vi "nanocal -- nuclear schottky goodness V2.vi"(0 "ζ":dbl(slide)=0.23496699999999998 min=0.0 max=0.3 step=1e-06 scale=0.01..10.0 scale format="%#_3p", 1 "T1":dbl(slide)=0.26762 min=0.0 max=0.3 step=1e-06 scale=0.001..10.0 scale format="%#_3p", 2 "τS":dbl(slide)=0.24445899999999998 min=0.0 max=0.3 step=1e-06 scale=0.001..10.0 scale format="%#_3p", 3 "τN":dbl(slide)=2.349673 min=0.0 max=0.3 step=1e-06 scale=0.001..10.0 scale format="%#_3p", 4 "τC":dbl(slide)=0.0059759999999999995 min=0.0 max=0.3 step=1e-06 scale=0.001..10.0 scale format="%#_3p", 5 "κ0":dbl(slide)=5.58e-10 min=0.0 max=0.3 step=1e-12 scale=1e-10..1e-06 scale format="%#_3p", 7 "ω (rad/sec)":dbl[](array[numeric])=[32012.991918577427, 32390.261658505893, 32466.39798177853, 32499.14340521798, 32517.39286113775, 32529.046092051318, 32537.14525712326, 32543.111142615544, 32547.696343954158, 32551.33675949651, 32554.302325209504, 32556.769142360055, 32558.856995237307, 32560.650202739795, 32562.209843476354, 32563.58125099723, 32564.7987833122, 32565.88895894197, 32566.872575330308, 32567.766175404246, 32568.583086316496, 32569.334166794306, 32570.02835688638, 32570.673085530187, 32571.274580490695, 32571.838104118455, 32572.36813539066, 32572.868514009202, 32573.342552524307, 32573.793126289274, 32574.222746575288, 32574.633618125405, 32575.027687968828, 32575.40668442971, 32575.772149741057, 32576.12546690325, 32576.467883345118, 32576.800529469096, 32577.124435064776, 32577.440543590797, 32577.749724325146, 32578.052781957467, 32578.35046682089, 32578.643482565894, 32578.932492128843, 32579.218126471686, 32579.500987779396, 32579.781656707495, 32580.06069600583, 32580.338656060805, 32580.616078519142, 32580.89350097748, 32581.171461032456, 32581.45050033079, 32581.73116925889, 32582.0140305666, 32582.29966469628, 32582.58867447239, 32582.88169000423, 32583.179375080817, 32583.48243271314, 32583.791613234323, 32584.10772197351, 32584.43162756919, 32584.764273480003, 32585.106690135035, 32585.460007297228, 32585.825472395412, 32586.204468856296, 32586.59853891288, 32587.009410462997, 32587.439030535847, 32587.889604513977, 32588.363642815923, 32588.86402143446, 32589.39405291983, 32589.957576334426, 32590.559071508098, 32591.203800151903, 32591.897990030815, 32592.64907072179, 32593.46598163404, 32594.359581707977, 32595.343197883154, 32596.433373726086, 32597.650906041054, 32599.022313348767, 32600.58195429849, 32602.375161800977, 32604.46301467823, 32606.929831615616, 32609.895397541775, 32613.535812870963, 32618.12101442274, 32624.086899701866, 32632.186064986967, 32643.839295900536, 32662.088751820305, 32694.834175046595, 32770.97049853239], 8 "weighting strategy":T1, 9 "Voltage IN (V)":cdb[](array[numeric])=[1.7183506006211996e-05+0.0i, 1.7124360968751133e-05+0.0i, 1.7049104347380084e-05+0.0i, 1.700437896335042e-05+0.0i, 1.6984579723285106e-05+0.0i, 1.702277369054923e-05+0.0i, 1.713094025845651e-05+0.0i, 1.734249707866828e-05+0.0i, 1.768320429215342e-05+0.0i, 1.8195281152538477e-05+0.0i, 1.8917228661806973e-05+0.0i, 1.9897834564883332e-05+0.0i, 2.154104046962704e-05+0.0i, 2.3247799321765792e-05+0.0i, 2.5364678450551808e-05+0.0i, 2.8645788781885885e-05+0.0i, 3.204749554800641e-05+0.0i, 3.783559691555022e-05+0.0i, 4.245015867332296e-05+0.0i, 4.909131821431355e-05+0.0i, 5.511821898441184e-05+0.0i, 6.178843506022867e-05+0.0i, 7.1079604965352e-05+0.0i, 7.922304381453334e-05+0.0i, 8.814778883893872e-05+0.0i, 9.806709148886077e-05+0.0i, 0.00011119043245647465+0.0i, 0.00012253184919712196+0.0i, 0.00013777724317049346+0.0i, 0.0001508081004573332+0.0i, 0.00016547294918783876+0.0i, 0.00018003847596605868+0.0i, 0.00019518361086534857+0.0i, 0.00021134179818259658+0.0i, 0.0002372041782935464+0.0i, 0.00025518143132024254+0.0i, 0.0002835129702467886+0.0i, 0.0003060118087631287+0.0i, 0.00032860772064336976+0.0i, 0.0003492674091322389+0.0i, 0.00037498324855458583+0.0i, 0.00040021078021115026+0.0i, 0.00041969942568205823+0.0i, 0.00044367338947118773+0.0i, 0.0004634793607238068+0.0i, 0.00047921028781215815+0.0i, 0.0004880906353641744+0.0i, 0.0004932212623741357+0.0i, 0.000491476456593048+0.0i, 0.000480893803992059+0.0i, 0.0004535995818650303+0.0i, 0.000417087772881063+0.0i, 0.0003564148692854789+0.0i, 0.0003049201646356487+0.0i, 0.00021260191240459413+0.0i, 0.00011714858948470126+0.0i, 1.675457544365132e-05+0.0i, -6.8674075405897e-05+0.0i, -0.000156473047607305+0.0i, -0.00026709373934749337+0.0i, -0.0003544271565676041+0.0i, -0.00047937600197311275+0.0i, -0.0006086290582260493+0.0i, -0.0007031877411848573+0.0i, -0.0007564526901441745+0.0i, -0.000802489180995596+0.0i, -0.0008414596018105983+0.0i, -0.0008809346482248761+0.0i, -0.0009073902840241921+0.0i, -0.0009264953054508651+0.0i, -0.0009405659412141811+0.0i, -0.000951649722530156+0.0i, -0.0009557485581057351+0.0i, -0.0009558464741053665+0.0i, -0.0009509110176922098+0.0i, -0.0009411315169847015+0.0i, -0.0009303400913929496+0.0i, -0.0009171113529290538+0.0i, -0.0009022111527275027+0.0i, -0.0008813746494947608+0.0i, -0.0008581837971946129+0.0i, -0.0008372063466683705+0.0i, -0.0008165626610594428+0.0i, -0.0007901155435838691+0.0i, -0.0007682834352800848+0.0i, -0.000746231015527196+0.0i, -0.0007238798463130141+0.0i, -0.0007015567569177018+0.0i, -0.000679301954671598+0.0i, -0.0006572001413831251+0.0i, -0.000629855254567978+0.0i, -0.0006083942229188815+0.0i, -0.0005768631156754208+0.0i, -0.0005562177438951648+0.0i, -0.0005359092039599222+0.0i, -0.0005145186443378148+0.0i, -0.0004951602053444319+0.0i, -0.00047624970229075174+0.0i, -0.0004577401041527736+0.0i, -0.00043519037796120065+0.0i], 11 "dz/dω IN (V)":cdb[](array[numeric])=[1.7183506006211996e-05+0.0i, 1.7124360968751133e-05+0.0i, 1.7049104347380084e-05+0.0i, 1.700437896335042e-05+0.0i, 1.6984579723285106e-05+0.0i, 1.702277369054923e-05+0.0i, 1.713094025845651e-05+0.0i, 1.734249707866828e-05+0.0i, 1.768320429215342e-05+0.0i, 1.8195281152538477e-05+0.0i, 1.8917228661806973e-05+0.0i, 1.9897834564883332e-05+0.0i, 2.154104046962704e-05+0.0i, 2.3247799321765792e-05+0.0i, 2.5364678450551808e-05+0.0i, 2.8645788781885885e-05+0.0i, 3.204749554800641e-05+0.0i, 3.783559691555022e-05+0.0i, 4.245015867332296e-05+0.0i, 4.909131821431355e-05+0.0i, 5.511821898441184e-05+0.0i, 6.178843506022867e-05+0.0i, 7.1079604965352e-05+0.0i, 7.922304381453334e-05+0.0i, 8.814778883893872e-05+0.0i, 9.806709148886077e-05+0.0i, 0.00011119043245647465+0.0i, 0.00012253184919712196+0.0i, 0.00013777724317049346+0.0i, 0.0001508081004573332+0.0i, 0.00016547294918783876+0.0i, 0.00018003847596605868+0.0i, 0.00019518361086534857+0.0i, 0.00021134179818259658+0.0i, 0.0002372041782935464+0.0i, 0.00025518143132024254+0.0i, 0.0002835129702467886+0.0i, 0.0003060118087631287+0.0i, 0.00032860772064336976+0.0i, 0.0003492674091322389+0.0i, 0.00037498324855458583+0.0i, 0.00040021078021115026+0.0i, 0.00041969942568205823+0.0i, 0.00044367338947118773+0.0i, 0.0004634793607238068+0.0i, 0.00047921028781215815+0.0i, 0.0004880906353641744+0.0i, 0.0004932212623741357+0.0i, 0.000491476456593048+0.0i, 0.000480893803992059+0.0i, 0.0004535995818650303+0.0i, 0.000417087772881063+0.0i, 0.0003564148692854789+0.0i, 0.0003049201646356487+0.0i, 0.00021260191240459413+0.0i, 0.00011714858948470126+0.0i, 1.675457544365132e-05+0.0i, -6.8674075405897e-05+0.0i, -0.000156473047607305+0.0i, -0.00026709373934749337+0.0i, -0.0003544271565676041+0.0i, -0.00047937600197311275+0.0i, -0.0006086290582260493+0.0i, -0.0007031877411848573+0.0i, -0.0007564526901441745+0.0i, -0.000802489180995596+0.0i, -0.0008414596018105983+0.0i, -0.0008809346482248761+0.0i, -0.0009073902840241921+0.0i, -0.0009264953054508651+0.0i, -0.0009405659412141811+0.0i, -0.000951649722530156+0.0i, -0.0009557485581057351+0.0i, -0.0009558464741053665+0.0i, -0.0009509110176922098+0.0i, -0.0009411315169847015+0.0i, -0.0009303400913929496+0.0i, -0.0009171113529290538+0.0i, -0.0009022111527275027+0.0i, -0.0008813746494947608+0.0i, -0.0008581837971946129+0.0i, -0.0008372063466683705+0.0i, -0.0008165626610594428+0.0i, -0.0007901155435838691+0.0i, -0.0007682834352800848+0.0i, -0.000746231015527196+0.0i, -0.0007238798463130141+0.0i, -0.0007015567569177018+0.0i, -0.000679301954671598+0.0i, -0.0006572001413831251+0.0i, -0.000629855254567978+0.0i, -0.0006083942229188815+0.0i, -0.0005768631156754208+0.0i, -0.0005562177438951648+0.0i, -0.0005359092039599222+0.0i, -0.0005145186443378148+0.0i, -0.0004951602053444319+0.0i, -0.00047624970229075174+0.0i, -0.0004577401041527736+0.0i, -0.00043519037796120065+0.0i]) -> (13 "G":dbl=-1.0, 14 "d ln G / d ln ζ":dbl=-1.0, 15 "d ln G / d ln τ1":dbl=-1.0, 16 "d ln G / d ln τS":dbl=-1.0, 17 "d ln G / d ln τN":dbl=-1.0, 18 "d ln G / d ln τC":dbl=-1.0, 19 "d ln G / d ln κ0":dbl=-1.0)   [LabVIEW 2020]
uses:
  nanocal-goodness-weighting-strategy.ctl
  3-lorentzian-heat-response action.ctl
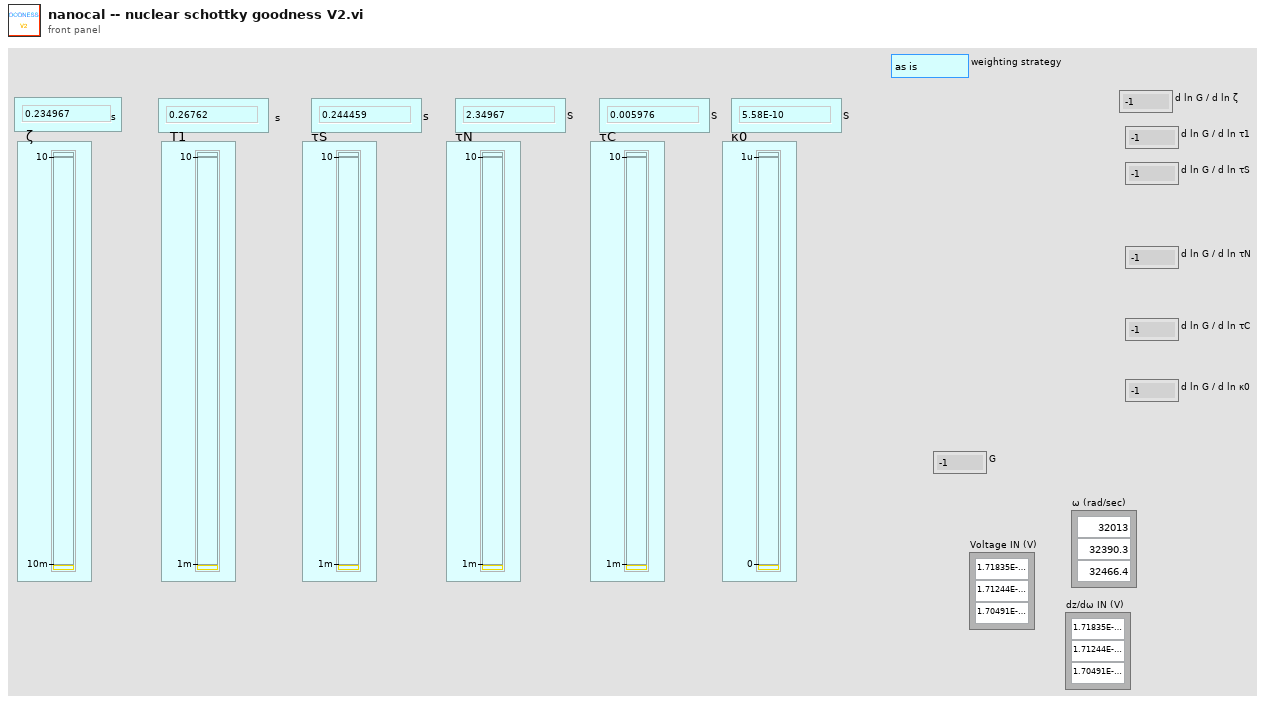
[diagram p1: front panel]
types:
  T1 = typedef "nanocal-goodness-weighting-strategy.ctl" = enum16{"as is", "|dz/dω|", "ω"}
  T2 = typedef "3-lorentzian-heat-response action.ctl" = enum16{"calc R", "create string", "calc m1m2m3", "dζ", "dT1", "dτS", "dτN", "dτC", "d-all", "dκ0"}
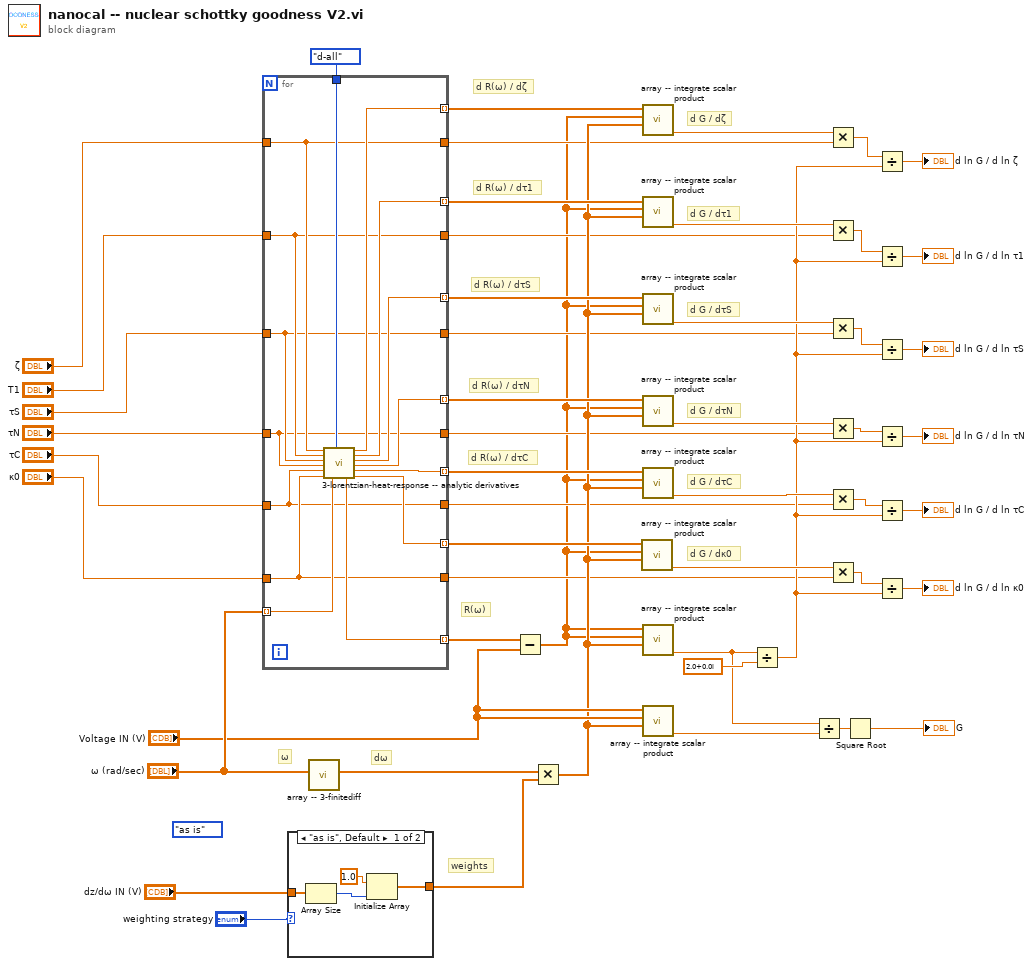
[diagram p0: block diagram]
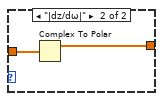
[diagram p2: hidden frame]
diagram:
  (unwired) nanocal-goodness-weighting-strategy."as is" ("action")
  # "weights"
  # "d G / dκ0"
  # "d G / dτC"
  # "d G / dτN"
  # "d G / dτS"
  # "d G / dτ1"
  # "d G / dζ"
  # "ω"
  # "d R(ω) / dτC"
  # "d R(ω) / dτN"
  # "d R(ω) / dτS"
  # "d R(ω) / dτ1"
  # "d R(ω) / dζ"
  # "R(ω)"
  # "dω"
  n1 = for {
    tunnel: "ζ" -> [w56]
    tunnel: "T1" -> [w55]
    tunnel: "τS" -> [w54]
    tunnel: "τN" -> [w53]
    tunnel: "τC" -> [w57]
    tunnel: "κ0" -> [w58]
    tunnel: 3-lorentzian-heat-response_action."d-all" ("action") -> [w64]
    tunnel: "ω (rad/sec)" -> [w67] mode=indexing
    tunnel: [w66] -> w51 mode=indexing
    tunnel: [w65] -> w33 mode=indexing
    tunnel: [w63] -> w31 mode=indexing
    tunnel: [w62] -> w29 mode=indexing
    tunnel: [w61] -> w27 mode=indexing
    tunnel: [w60] -> w25 mode=indexing
    tunnel: [w59] -> w23 mode=indexing
    tunnel: [w58] -> w10
    tunnel: [w57] -> w8
    tunnel: [w56] -> w7
    tunnel: [w55] -> w6
    tunnel: [w54] -> w5
    tunnel: [w53] -> w4
    n2 = call "3-lorentzian-heat-response -- analytic derivatives.vi"("ζ"=w56, "T1"=w55, "τS"=w54, "τN"=w53, "τC"=w57, "κ0"=w58, "ω (rad/sec)"=w67, "action"=w64) -> ("R(ω)"=w66:cdb, "d R(ω) / dζ"=w65:cdb, "d R(ω) /  dT1"=w63:cdb, "d R(ω) /  d τS"=w62:cdb, "d R(ω) /  d τN"=w61:cdb, "d R(ω) /  d τC"=w60:cdb, "d R(ω) /  d κ0"=w59:cdb)  [unwired: 5 in]
  }
  n3 = case shown="\"as is\", Default" "weighting strategy" {
    tunnel: [w68 w72] -> w3
    tunnel: "dz/dω IN (V)" -> [w70 w73]
    frame "as is", Default {
      n4 = Array Size(array=w70) -> (size(s)=w71:i32)
      n5 = Initialize Array(1.0 ("element"), w71) -> (w68:dbl[])
    }
    frame "|dz/dω|" {
      n6 = Complex To Polar(r * e^(i*theta)=w73) -> (r=w72:dbl[])  [unwired: 1 out]
    }
  }
  n7 = call "array -- 3-finitediff.vi"("ω (rad/sec)"="ω (rad/sec)") -> ("dω (rad/sec)"=w18:cdb[])  [unwired: 10 in]
  n8 = Subtract(x=w51, y="Voltage IN (V)") -> (x-y=w2:cdb[])
  n9 = Multiply(x=w18, y=w3) -> (x*y=w14:cdb[])
  n10 = call "array -- integrate scalar product.vi"("dω"=w14, "B"=w2, "A"=w23) -> ("total"=w22:cdb)  [unwired: 7 in, 1 out]
  n11 = call "array -- integrate scalar product.vi"("dω"=w14, "B"=w2, "A"=w33) -> ("total"=w32:cdb)  [unwired: 7 in, 1 out]
  n12 = call "array -- integrate scalar product.vi"("dω"=w14, "B"=w2, "A"=w31) -> ("total"=w30:cdb)  [unwired: 7 in, 1 out]
  n13 = call "array -- integrate scalar product.vi"("dω"=w14, "B"=w2, "A"=w29) -> ("total"=w28:cdb)  [unwired: 7 in, 1 out]
  n14 = call "array -- integrate scalar product.vi"("dω"=w14, "B"=w2, "A"=w27) -> ("total"=w26:cdb)  [unwired: 7 in, 1 out]
  n15 = call "array -- integrate scalar product.vi"("dω"=w14, "B"=w2, "A"=w25) -> ("total"=w24:cdb)  [unwired: 7 in, 1 out]
  n16 = call "array -- integrate scalar product.vi"("dω"=w14, "B"=w2, "A"=w2) -> ("total"=w13:cdb)  [unwired: 7 in, 1 out]
  n17 = call "array -- integrate scalar product.vi"("dω"=w14, "B"="Voltage IN (V)", "A"="Voltage IN (V)") -> ("total"=w12:cdb)  [unwired: 7 in, 1 out]
  n18 = Divide(x=w13, y=cdb 2.0+0.0i) -> (x/y=w20:cdb)
  n19 = Divide(x=w13, y=w12) -> (x/y=w19:cdb)
  n20 = Multiply(x=w32, y=w7) -> (x*y=w50:cdb)
  n21 = Multiply(x=w30, y=w6) -> (x*y=w47:cdb)
  n22 = Multiply(x=w28, y=w5) -> (x*y=w44:cdb)
  n23 = Multiply(x=w26, y=w4) -> (x*y=w41:cdb)
  n24 = Multiply(x=w24, y=w8) -> (x*y=w38:cdb)
  n25 = Multiply(x=w22, y=w10) -> (x*y=w36:cdb)
  n26 = Square Root(x=w19) -> (sqrt(x)=→"G":cdb)
  n27 = Divide(x=w50, y=w20) -> (x/y=→"d ln G / d ln ζ":cdb)
  n28 = Divide(x=w47, y=w20) -> (x/y=→"d ln G / d ln τ1":cdb)
  n29 = Divide(x=w44, y=w20) -> (x/y=→"d ln G / d ln τS":cdb)
  n30 = Divide(x=w41, y=w20) -> (x/y=→"d ln G / d ln τN":cdb)
  n31 = Divide(x=w38, y=w20) -> (x/y=→"d ln G / d ln τC":cdb)
  n32 = Divide(x=w36, y=w20) -> (x/y=→"d ln G / d ln κ0":cdb)
